vi "ParseArguments.vi"(8 "error in (no error)":errorcluster, 10 "Inputs":string[](array[string]), 11 "ExecuteBuildSpec in":refnum<class "ExecuteBuildSpec.lvclass">) -> (0 "error out":errorcluster, 3 "ExecuteBuildSpec out":refnum<class "ExecuteBuildSpec.lvclass">)   [LabVIEW 2014, in "ExecuteBuildSpec.lvclass"]
uses:
  ExecuteBuildSpec.lvclass
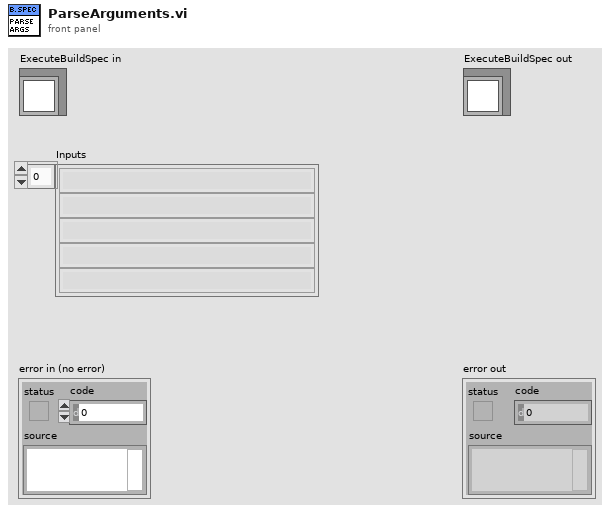
[diagram p1: front panel]
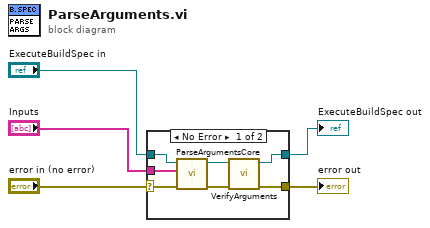
[diagram p0: block diagram]
diagram:
  n1 = case shown="No Error" "error in (no error)" {
    selector: "error in (no error)" -> [w11 w14]
    tunnel: [w7 w14] -> w4
    tunnel: "ExecuteBuildSpec in" -> [w12 w13]
    tunnel: [w6 w13] -> w2
    tunnel: "Inputs" -> [w10 _]
    frame No Error {
      n2 = call "ParseArgumentsCore.vi"("error in (no error)"=w11, "Inputs"=w10, "ExecuteBuildSpec in"=w12) -> ("error out"=w8:errorcluster, "ExecuteBuildSpec out"=w9:refnum<class "ExecuteBuildSpec.lvclass">)  [unwired: 7 in]
      n3 = call "VerifyArguments.vi"("error in (no error)"=w8, "ExecuteBuildSpec in"=w9) -> ("error out"=w7:errorcluster, "ExecuteBuildSpec out"=w6:refnum<class "ExecuteBuildSpec.lvclass">)  [unwired: 8 in]
    }
    frame Error {
    }
  }
  "error out" <- w4
  "ExecuteBuildSpec out" <- w2
